vi "PID_2Chan_V2.vi"() -> ()   [LabVIEW 2016]
uses:
  <vilib>/Analysis/baseanly.llb/Mean (DBL).vi
  <vilib>/addons/control/pid/pid.llb/PID Advanced (DBL Array).vi
  <vilib>/addons/control/pid/pid.llb/PID Parameter Manager (DBL Array).vi
  <vilib>/addons/control/pid/pid.llb/PID Derivative Action Buffered (DBL Array).vi
  <vilib>/addons/control/pid/pid.llb/PID Get Advanced Error (DBL Array).vi
  <vilib>/addons/control/pid/pid.llb/PID Integral Action Buffered (DBL Array).vi
  <vilib>/addons/control/pid/pid.llb/PID Resize 1D Array.vi
  <vilib>/addons/control/pid/pid.llb/PID Get Advanced Error (DBL).vi
  <userlib>/Fluigent/Fluigent MFCS/FluigentMFCS_Full.llb/MFCS_EZ Detect.vi
  <userlib>/Fluigent/Fluigent MFCS/FluigentMFCS_Full.llb/MFCS_EZ Initialization.vi
  <userlib>/Fluigent/Fluigent MFCS/FluigentMFCS_Full.llb/MFCS_EZ Write Channel Pressure.vi
  <userlib>/Fluigent/Fluigent MFCS/FluigentMFCS_Full.llb/MFCS_EZ Close.vi
  <vilib>/addons/control/pid/NI_PID_pid.lvlib
  <vilib>/Analysis/NI_AALBase.lvlib
panel:
  in  "reset Averging":bool
  in  "Values to Display":dbl=400.0
  in  "Sec2wait":dbl
  in  "Set current Pressure to manual pressure":bool
  out "Pressures":cluster{"[0]":dbl, "[1]":dbl}(graph)={"[0]"=667.158203125, "[1]"=642.5421752929688}
  out "Flow Rates":dbl[](array[numeric])=[210.22133042674415, 339.55476284846253]
  out "Err Signal":cluster{"[0]":dbl, "[1]":dbl, "[2]":dbl}(graph)={"[0]"=0.010223906724793324, "[1]"=0.010666567578281615, "[2]"=0.0}
  in  "stop":bool=TRUE
  out "Flow Rates":T1(graph)={"appended array[0]"=210.22133042674415, "appended array[1]"=339.55476284846253}
  in  "Valves":enum16{"1", "2", "3", "4", "5", "6", "7", "8"}[](array[ring])=[enum."6", enum."7"]
  in  "Pressure Channels":i16[](array[numeric])=[2, 3]
  in  "Manual Pressure Set":dbl[](array[numeric])=[581.6619074041193, 548.1519459117543]
  in  "PID On":bool=TRUE
  in  "reinitialize? (F)":bool
  in  "F0 Setpoint":dbl=350.0
  in  "F1 Setpoint":dbl=210.0
  in  "PID Gains":T2(array[cluster])=[{"Proportional Gain"=1.0, "Integral Time"=1.0, "Derivative Time"=0.0}, {"Proportional Gain"=1.5, "Integral Time"=1.0, "Derivative Time"=0.0}]
  in  "Add Ctrl?":bool
  in  "Boards":enum16{"A", "B", "C"}[](array[ring])=[enum."A", enum."A"]
  in  "Valves":enum16{"1", "2", "3", "4", "5", "6", "7", "8"}[](array[ring])=[enum."5", enum."4"]
  # "Differential"
  # "Tonic"
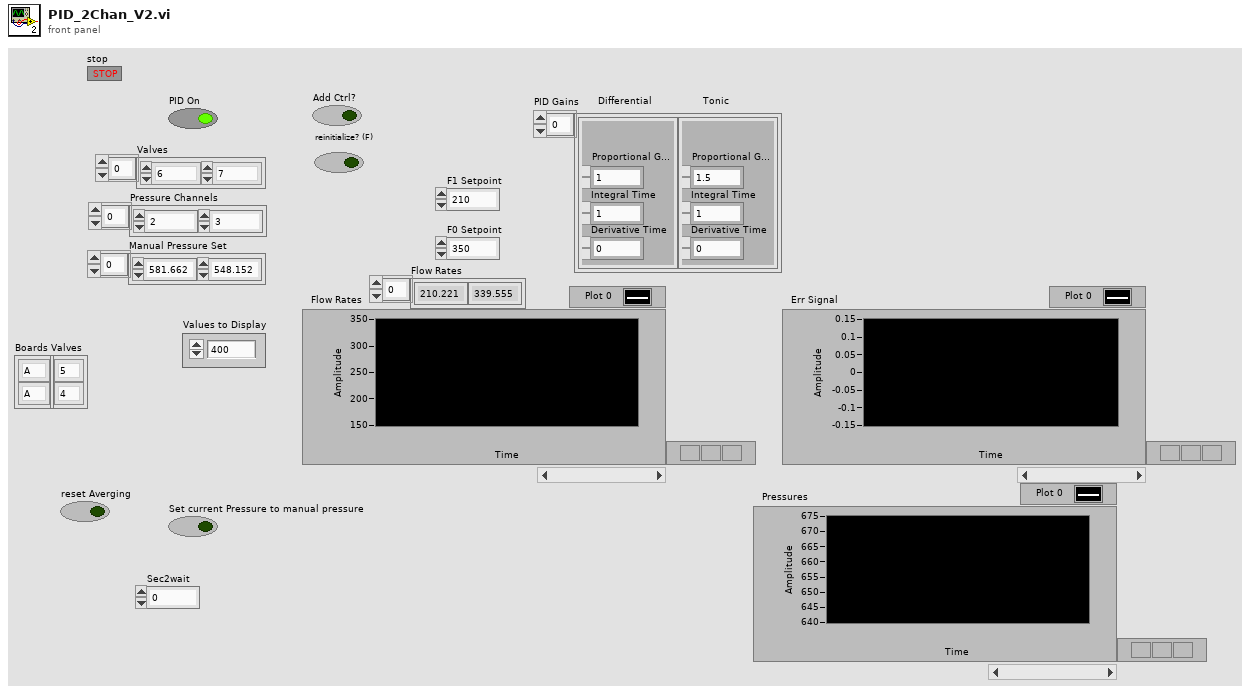
[diagram p1: front panel]
types:
  T1 = cluster{"appended array[0]":dbl, "appended array[1]":dbl}
  T2 = cluster{"Proportional Gain":dbl, "Integral Time":dbl, "Derivative Time":dbl}[]
  T3 = typedef "_EZmfcsSN.ctl" = u16
  T4 = typedef "_EZmfcsRefNum.ctl" = refnum<k1>
  T5 = cluster{"setpoint high":dbl, "setpoint low":dbl}[]
  T6 = cluster{"Proportional Gain":dbl, "Integral Time":dbl, "Derivative Time":dbl}
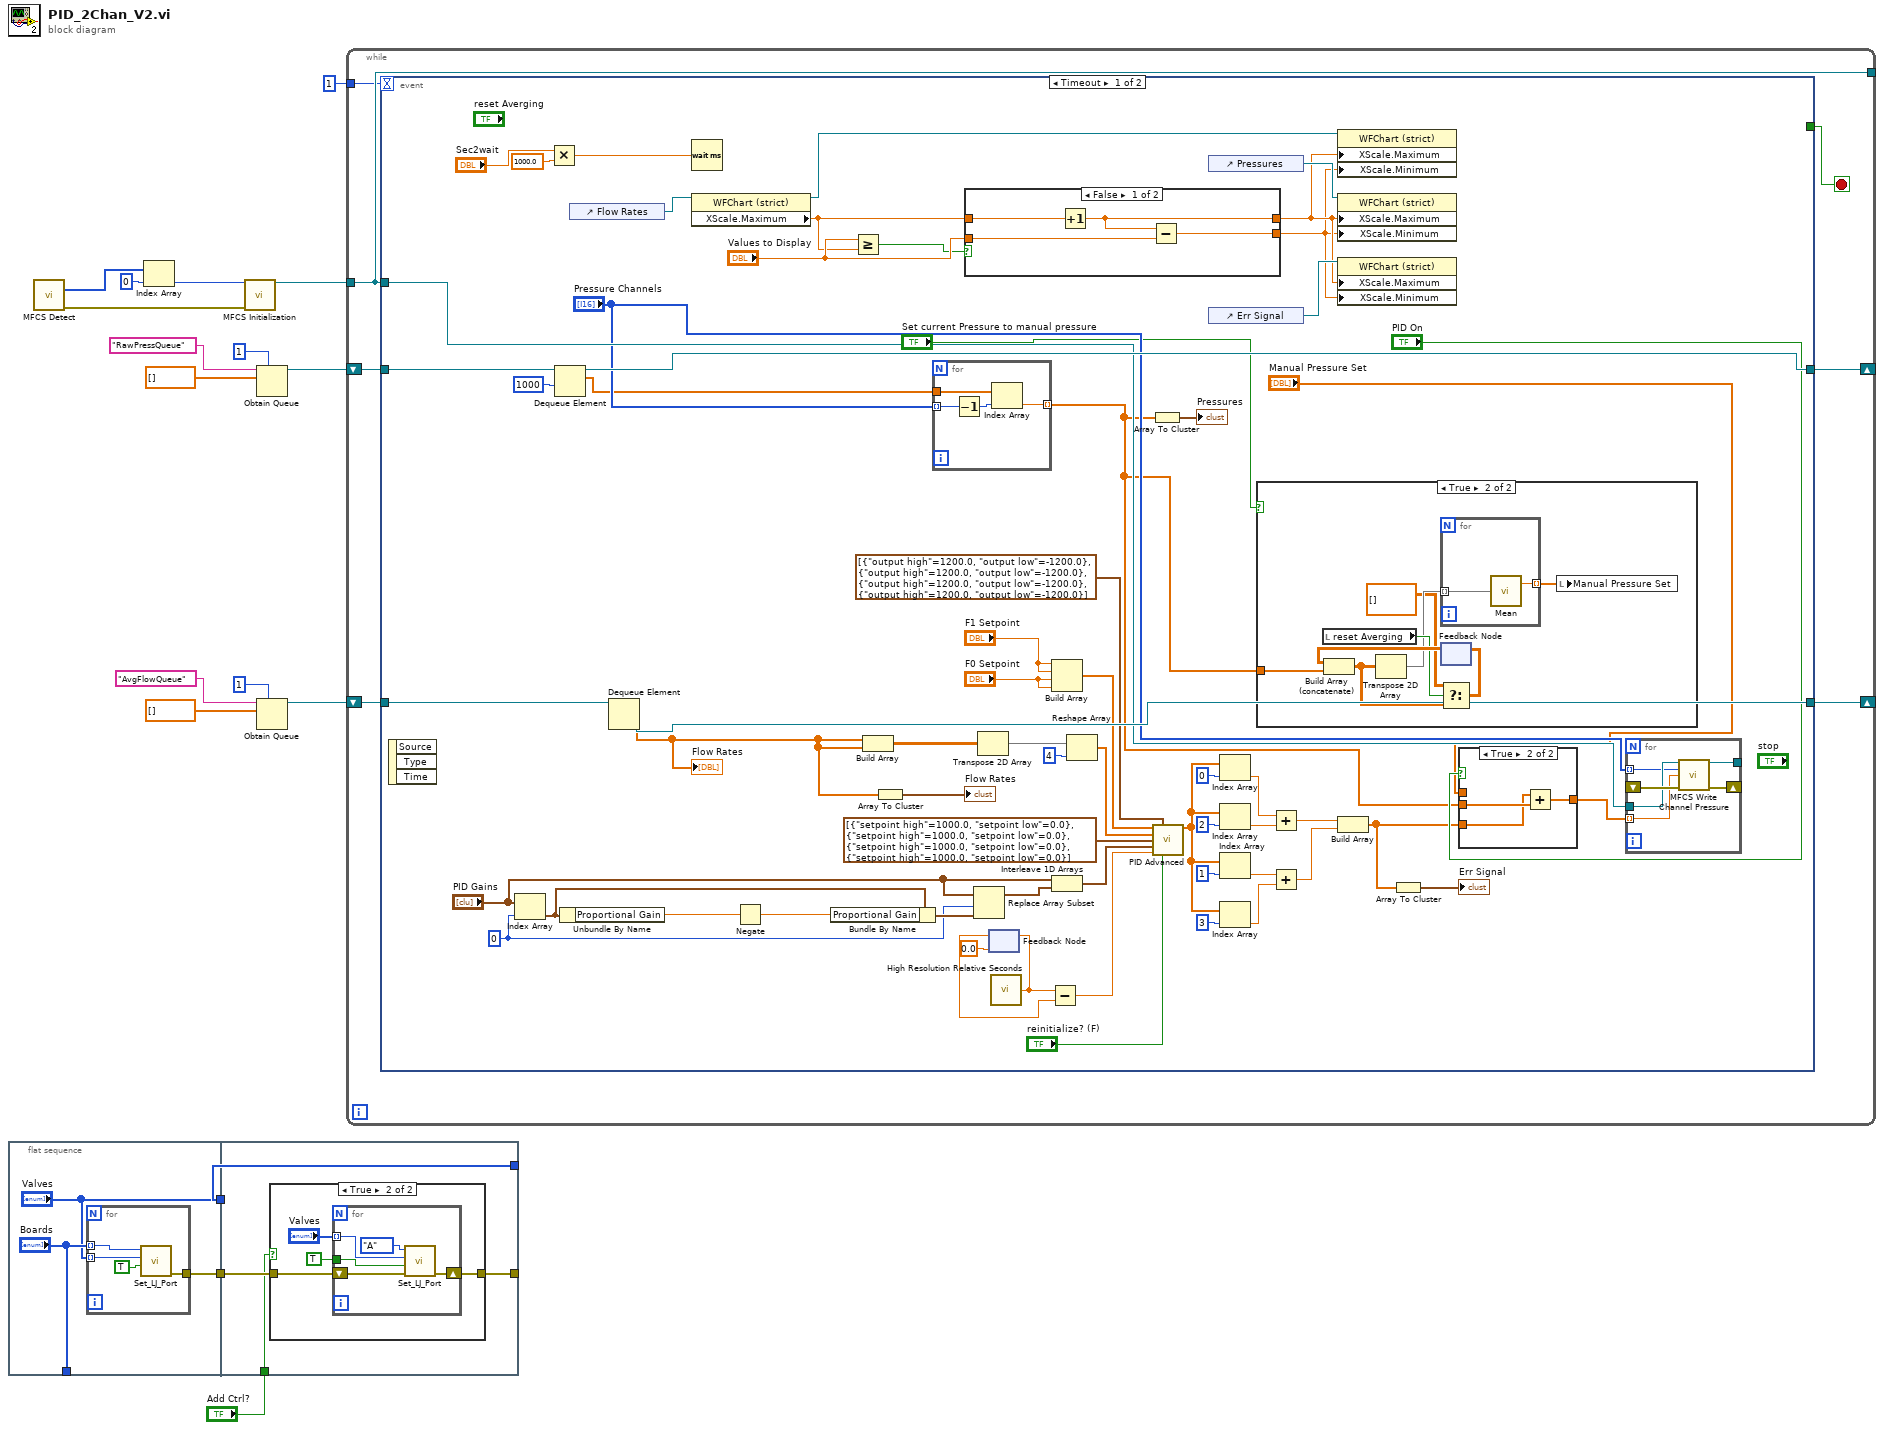
[diagram p0: block diagram]
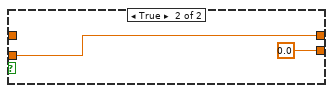
[diagram p3: hidden frame]
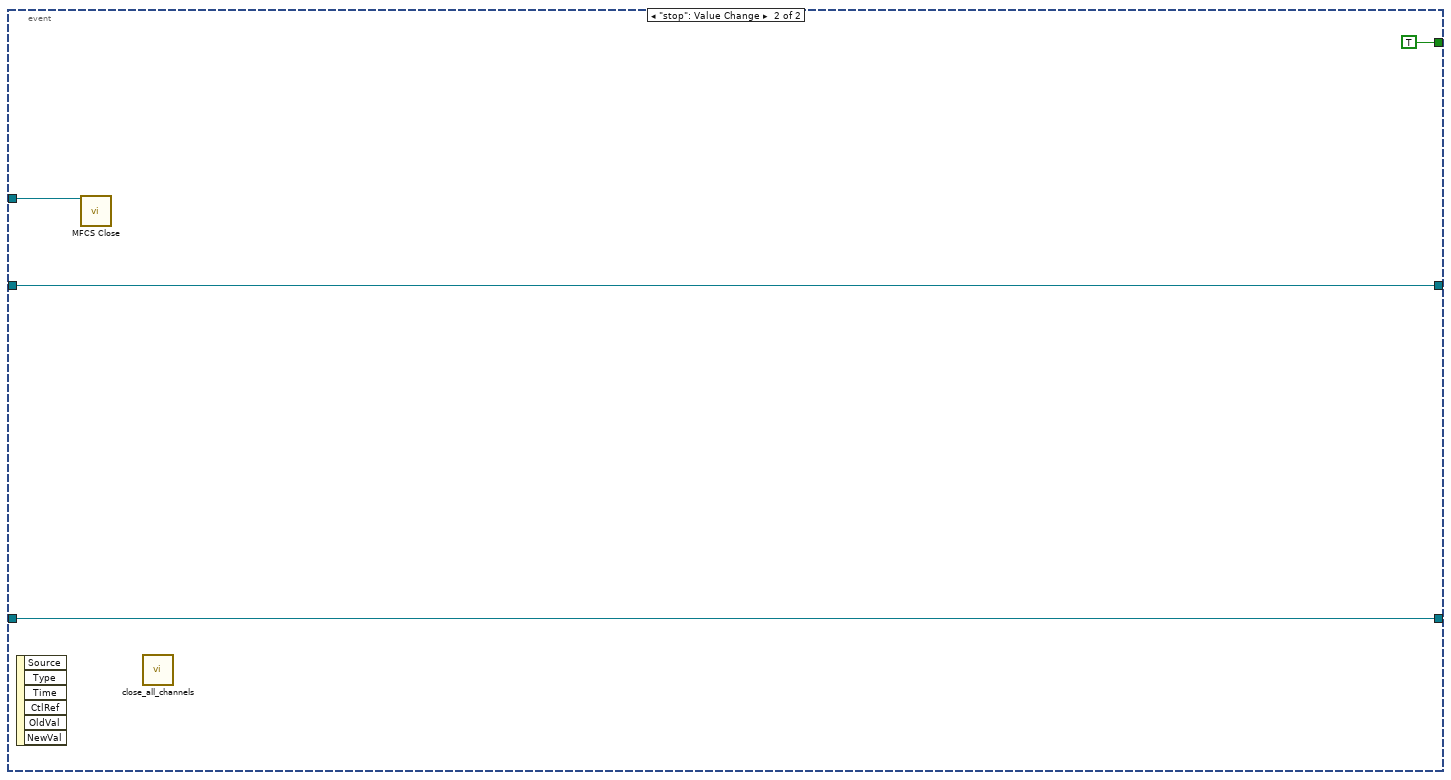
[diagram p5: hidden frame]
diagram:
  n1 = flat-sequence {
    tunnel: ["Boards"] -> _
    tunnel: [w20] -> w17
    tunnel: ["Valves"] -> w16
    tunnel: [w28] -> _
    tunnel: [w26] -> _
    tunnel: w17 -> [w27]
    tunnel: w16 -> [w28]
    tunnel: "Add Ctrl?" -> [w25]
    frame #0 {
      n2 = for {
        tunnel: "Valves" -> [w24] mode=indexing
        tunnel: "Boards" -> [w23] mode=indexing
        tunnel: [w21] -> w20
        n3 = call "Set_LJ_Port.vi"("State"=TRUE, "Channel"=w24, "Flowboard"=w23) -> ("error out"=w21:errorcluster)  [unwired: 8 in]
      }
    }
    frame #1 {
      n4 = case shown="True" w25 {
        tunnel: w27 -> [w29 w33]
        tunnel: [w29 w32] -> w26
        frame False {
        }
        frame True {
          n5 = for {
            tunnel: TRUE ("State") -> [w36]
            shift-right: [w37] -> w32
            shift-left: w33 -> [w38]
            tunnel: "Valves" -> [w35] mode=indexing
            n6 = call "Set_LJ_Port.vi"("error in"=w38, "State"=w36, "Channel"=w35, "Flowboard"=enum16{"A", "B", "C"}."A") -> ("error out"=w37:errorcluster)  [unwired: 7 in]
          }
        }
      }
    }
  }
  n7 = call-poly <userlib>:"MFCS Detect.vi"() -> ("[SN MFCS_EZ]"=w14:T3[], "error out"=w12:errorcluster)  [unwired: 14 in]
  n8 = Index Array(array=w14, index=0) -> (element=w13:T3)
  n9 = call-poly <userlib>:"MFCS Initialization.vi"("SN MFCS_EZ"=w13, "error in (no error)"=w12) -> ("MFCS_EZ"=w10:T4)  [unwired: 11 in, 2 out]
  n10 = Obtain Queue(max queue size (-1, unlimited)=1, name (unnamed)="RawPressQueue", element data type=dbl[] [] ("appended array")) -> (queue out=w2:refnum<queue>)  [unwired: 2 in, 2 out]
  n11 = Obtain Queue(max queue size (-1, unlimited)=1, name (unnamed)="AvgFlowQueue", element data type=dbl[] [] ("appended array")) -> (queue out=w3:refnum<queue>)  [unwired: 2 in, 2 out]
  n12 = while {
    tunnel: [w41] -> _
    tunnel: w10 -> [w41]
    shift-right: [w43] -> _
    shift-left: w2 -> [w44]
    shift-right: [w42] -> _
    shift-left: w3 -> [w45]
    tunnel: 1 -> [w39]
    stop <- w40 stop-if-true
    n13 = event shown="[0] Timeout" {
      selector: _ -> [_ _]
      dyn-events: _ -> [_ _]
      timeout: w39 -> [_ _]
      tunnel: w45 -> [w108 w139]
      tunnel: w44 -> [w107 w140]
      tunnel: [w106 w140] -> w43
      tunnel: [w105 w139] -> w42
      tunnel: w41 -> [w86 w141]
      tunnel: [_ TRUE] -> w40
      event Timeout {
        w60 = 0 ("index")
        n14 = event-data() -> ()  [unwired: 1 in, 3 out]
        n15 = Index Array(array="PID Gains", index=w60) -> (element=w64:T6)
        n16 = Multiply(x="Sec2wait", y=1000.0) -> (x*y=w67:dbl)
        n17 = Dequeue Element(queue=w107, timeout in ms (-1)=1000) -> (queue out=w106:refnum<queue>, element=w71:dbl[])  [unwired: 1 in, 2 out]
        n18 = Unbundle By Name(w64) -> ("Proportional Gain"=w65:dbl)
        n19 = control-ref of="Flow Rates"() -> (w53:refnum<vi>)
        n20 = Dequeue Element(queue=w108) -> (queue out=w105:refnum<queue>, element=w55:dbl[])  [unwired: 2 in, 2 out]
        "Flow Rates" <- w55
        n21 = Wait (ms)(milliseconds to wait=w67) -> ()  [unwired: 1 out]
        n22 = property on="Property Node" class="WFChart (strict)"(reference=w53) -> (reference out=w52:refnum<vi>, "XScale.Maximum"=w56:dbl)  [unwired: 1 in, 1 out]
        n23 = Negate(x=w65) -> (-x=w63:dbl)
        n24 = Bundle By Name(cluster=w64, "Proportional Gain"=w63) -> (w61:T6)
        n25 = Greater Or Equal?(x="Values to Display", y=w56) -> (x >= y?=w57:bool)
        n26 = Build Array(w55, w55) -> (w89:dbl[][])
        n27 = Array To Cluster(array=w55) -> (cluster=→"Flow Rates":T1)
        n28 = for {
          tunnel: "Pressure Channels" -> [w128] mode=indexing
          tunnel: w71 -> [w127]
          tunnel: [w125] -> w46 mode=indexing
          n29 = Decrement(x=w128) -> (x-1=w126:i16)
          n30 = Index Array(array=w127, index=w126) -> (element=w125:dbl)
        }
        n31 = case shown="False" w57 {
          tunnel: "Values to Display" -> [w120 w124]
          tunnel: w56 -> [w122 _]
          tunnel: [w119 w124] -> w49
          tunnel: [w121 0.0] -> w48
          frame False {
            n32 = Increment(x=w122) -> (x+1=w119:dbl)
            n33 = Subtract(x=w119, y=w120) -> (x-y=w121:dbl)
          }
          frame True {
          }
        }
        n34 = Replace Array Subset(array="PID Gains", new element=w61, index=w60) -> (w59:T2)
        n35 = Transpose 2D Array(2D array=w89) -> (transposed array=w76:dbl[][])
        n36 = feedback #1(0.0 ("relative seconds")) -> (w83:dbl)
        n37 = call <vilib>:"High Resolution Relative Seconds.vi"() -> ("relative seconds"=w82:dbl)
        n38 = feedback-in #1(w82) -> ()
        n39 = Subtract(x=w82, y=w83) -> (x-y=w81:dbl)
        n40 = Build Array("F1 Setpoint", "F1 Setpoint", "F0 Setpoint", "F0 Setpoint") -> (w91:dbl[])
        n41 = Interleave 1D Arrays("PID Gains", w59) -> (w66:T2)
        n42 = Reshape Array(w76, 4 ("dimension size")) -> (w88:dbl[])
        n43 = Array To Cluster(array=w46) -> (cluster=→"Pressures":cluster{"[0]":dbl, "[1]":dbl})
        n44 = call-poly <vilib>:"PID Advanced.vi"("setpoint"=w91, "output range"=cluster{"output high":dbl, "output low":dbl}[] [{"output high"=1200.0, "output low"=-1200.0}, {"output high"=1200.0, "output low"=-1200.0}, {"output high"=1200.0, "output low"=-1200.0}, {"output high"=1200.0, "output low"=-1200.0}], "process variable"=w88, "setpoint range"=T5 [{"setpoint high"=1000.0, "setpoint low"=0.0}, {"setpoint high"=1000.0, "setpoint low"=0.0}, {"setpoint high"=1000.0, "setpoint low"=0.0}, {"setpoint high"=1000.0, "setpoint low"=0.0}], "PID gains"=w66, "dt (s)"=w81, "reinitialize? (F)"="reinitialize? (F)") -> ("output"=w92:dbl[])  [unwired: 7 in, 1 out]
        n45 = control-ref of="Pressures"() -> (w51:refnum<vi>)
        n46 = control-ref of="Err Signal"() -> (w50:refnum<vi>)
        n47 = Index Array(array=w92, index=0) -> (element=w98:dbl)
        n48 = Index Array(array=w92, index=2) -> (element=w97:dbl)
        n49 = Index Array(array=w92, index=1) -> (element=w96:dbl)
        n50 = Index Array(array=w92, index=3) -> (element=w95:dbl)
        n51 = case shown="True" "Set current Pressure to manual pressure" {
          tunnel: w46 -> [_ w109]
          frame False {
          }
          frame True {
            n52 = local read "reset Averging"() -> (w115:bool)
            n53 = feedback #2() -> (w116:dbl[][])  [unwired: 1 in]
            n54 = Build Array (concatenate)(w116, w109) -> (w112:dbl[][])
            n55 = Transpose 2D Array(2D array=w112) -> (transposed array=w114:dbl[][])
            n56 = for {
              tunnel: w114 -> [w118] mode=indexing
              tunnel: [w117] -> w110 mode=indexing
              n57 = call-poly <vilib>:"Mean.vi"("X"=w118) -> ("mean"=w117:dbl)  [unwired: 1 out]
            }
            n58 = Select(t=dbl[][] [] ("appended array"), s=w115, f=w112) -> (s? t:f=w111:dbl[][])
            n59 = feedback-in #2(w111) -> ()
            n60 = local write "Manual Pressure Set"(w110) -> ()
          }
        }
        n61 = Add(x=w98, y=w97) -> (x+y=w94:dbl)
        n62 = Add(x=w96, y=w95) -> (x+y=w93:dbl)
        n63 = property on="Property Node" class="WFChart (strict)"(reference=w52, "XScale.Maximum"=w49, "XScale.Minimum"=w48) -> ()  [unwired: 1 in, 2 out]
        n64 = property on="Property Node" class="WFChart (strict)"(reference=w51, "XScale.Maximum"=w49, "XScale.Minimum"=w48) -> ()  [unwired: 1 in, 2 out]
        n65 = property on="Property Node" class="WFChart (strict)"(reference=w50, "XScale.Maximum"=w49, "XScale.Minimum"=w48) -> ()  [unwired: 1 in, 2 out]
        n66 = Build Array(w94, w93) -> (w75:dbl[])
        n67 = Array To Cluster(array=w75) -> (cluster=→"Err Signal":cluster{"[0]":dbl, "[1]":dbl, "[2]":dbl})
        n68 = case shown="True" "PID On" {
          tunnel: "Manual Pressure Set" -> [w129 _]
          tunnel: w75 -> [_ w131]
          tunnel: w46 -> [_ w132]
          tunnel: [w129 w130] -> w79
          frame False {
          }
          frame True {
            n69 = Add(x=w131, y=w132) -> (x+y=w130:dbl[])
          }
        }
        n70 = for {
          shift-right: [w137] -> _
          shift-left: _ -> [w138]
          tunnel: [w136] -> _
          tunnel: w86 -> [w135]
          tunnel: w79 -> [w134] mode=indexing
          tunnel: "Pressure Channels" -> [w133] mode=indexing
          n71 = call-poly <userlib>:"MFCS Write Channel Pressure.vi"("MFCS_EZ"=w135, "Channel Number (default=1)"=w133, "Pressure (mBar)"=w134, "error in (no error)"=w138) -> ("MFCS_EZ out"=w136:T4, "error out"=w137:errorcluster)  [unwired: 10 in]
        }
      }
      event "stop": Value Change {
        n72 = event-data() -> ()  [unwired: 1 in, 6 out]
        n73 = call-poly <userlib>:"MFCS Close.vi"("MFCS_EZ"=w141) -> ()  [unwired: 14 in, 1 out]
        n74 = call "close_all_channels.vi"() -> ()  [unwired: 12 in]
      }
    }
  }
